vi "TEST22.vi"(8 "error in (no error)":errorcluster) -> (0 "error out":errorcluster)   [LabVIEW 2019]
panel:
  in  "Boolean":bool
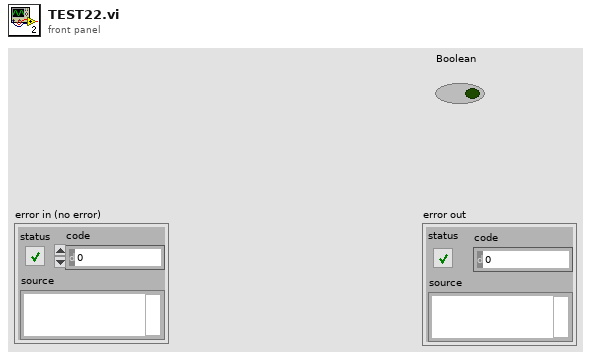
[diagram p1: front panel]
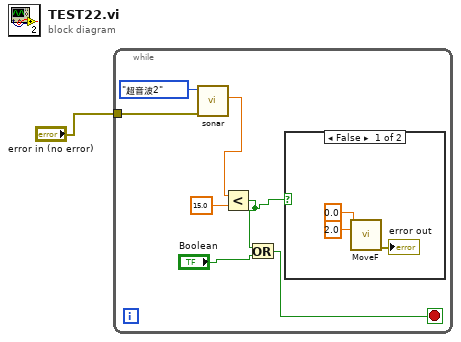
[diagram p0: block diagram]
diagram:
  n1 = while {
    tunnel: "error in (no error)" -> [w3]
    stop <- w6 stop-if-true
    n2 = call "sonar.vi"("error in (no error)"=w3, "選擇超音波"=enum16{"請選擇超音波", "超音波1", "超音波2", "超音波3", "超音波4"}."超音波2") -> ("公分"=w5:dbl)  [unwired: 8 in, 1 out]
    n3 = Less?(x=w5, y=15.0) -> (x < y?=w4:bool)
    n4 = Or(x=w4, y="Boolean") -> (x .or. y?=w6:bool)
    n5 = case shown="False" w4 {
      frame False {
        n6 = call "MoveF.vi"("X"=0.0, "Y"=2.0) -> ("error out"=→"error out":errorcluster)  [unwired: 13 in]
      }
      frame True {
      }
    }
  }
